vi "Plot Label StringToNum.vi"(7 "Format String":string) -> (3 "Hide trailing zeros":bool, 4 "Digit Type":i32, 6 "just/pad":i32(ring) items=["Pad with spaces on left", "Pad with spaces on right", "Pad with zeros on left"], 8 "Minimum Field Width":i32, 10 "Digits of Precision":i32, 14 "exponent":bool, 15 "Numeric Format":i32)   [LabVIEW 2020, in "3D Plot.lvclass"]
uses:
  <vilib>/Math Plots/3D Math Plots/3D Plot/3D Plot/3D Plot.lvclass
panel:
  out "Modifiers":string
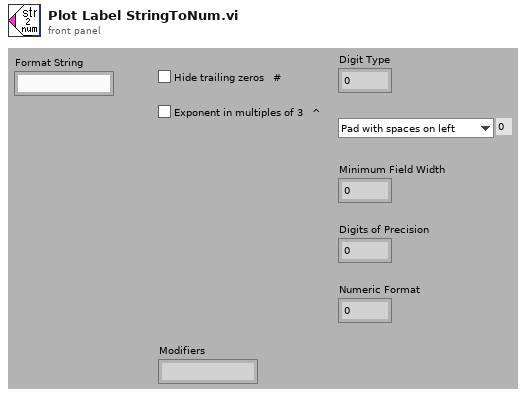
[diagram p1: front panel]
types:
  T1 = cluster{"Code Char":string, "Precision":i32, "MinWidth":u16, "EmbeddedString":string, "Modifiers":string}
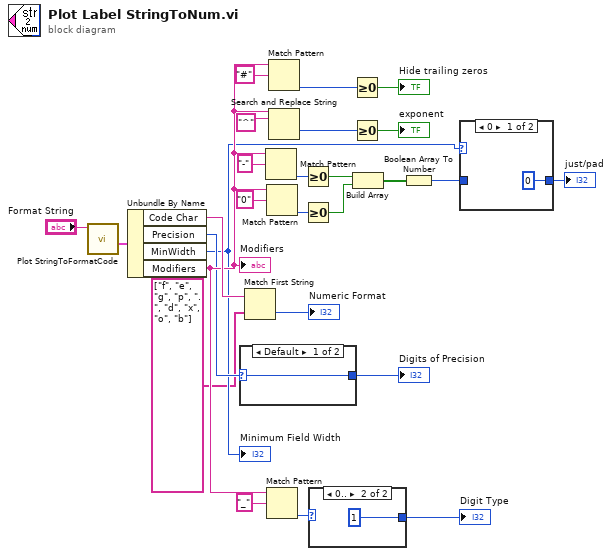
[diagram p0: block diagram]
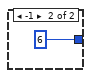
[diagram p3: hidden frame]
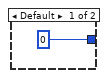
[diagram p4: hidden frame]
diagram:
  n1 = call <vilib>:"Plot StringToFormatCode.vi"("Start String"="Format String") -> ("FormatCode"=w25:T1)  [unwired: 10 out]
  n2 = Unbundle By Name(w25) -> ("Code Char"=w24:string, "Precision"=w6:i32, "MinWidth"=w4:u16, "Modifiers"=w11:string)
  "Minimum Field Width" <- w4
  "Modifiers" <- w11
  n3 = case shown="Default" w6 {
    selector: w6 -> [w28 _]
    tunnel: [w28 6] -> w5
    frame Default {
    }
    frame -1 {
    }
  }
  "Digits of Precision" <- w5
  n4 = Match First String(2:string[] ["f", "e", "g", "p", ".", "d", "x", "o", "b"] ("formats"), 3:w24) -> (0:→"Numeric Format":i32)  [unwired: 1 out]
  n5 = Match Pattern(string=w11, regular expression="-") -> (offset past match=w14:i32)  [unwired: 4 out]
  n6 = Match Pattern(string=w11, regular expression="0") -> (offset past match=w13:i32)  [unwired: 4 out]
  n7 = Match Pattern(string=w11, regular expression="_") -> (offset past match=w22:i32)  [unwired: 4 out]
  n8 = Match Pattern(string=w11, regular expression="#") -> (offset past match=w19:i32)  [unwired: 4 out]
  n9 = Search and Replace String(input string=w11, search string="^") -> (offset past replacement=w9:i32)  [unwired: 1 in, 8 out]
  n10 = Greater Or Equal To 0?(x=w14) -> (x >= 0?=w7:bool)
  n11 = Greater Or Equal To 0?(x=w13) -> (x >= 0?=w8:bool)
  n12 = case shown="0.." w22 {
    tunnel: [0 1] -> w21
    frame Default {
    }
    frame 0.. {
    }
  }
  "Digit Type" <- w21
  n13 = Greater Or Equal To 0?(x=w19) -> (x >= 0?=→"Hide trailing zeros":bool)
  n14 = Greater Or Equal To 0?(x=w9) -> (x >= 0?=→"exponent":bool)
  n15 = Build Array(w7, w8) -> (w12:bool[])
  n16 = Boolean Array To Number(Boolean array=w12) -> (number=w3:u32)
  n17 = case shown="0" w4 {
    tunnel: w3 -> [_ w33]
    tunnel: [u32 0 w33] -> w2
    frame 0 {
    }
    frame Default {
    }
  }
  "just/pad" <- w2
